vi "Read AllowUndefinedNames.vi"(9 "VisaResourceName in":refnum<class "VisaResourceName.lvclass">) -> (3 "VisaResourceName out":refnum<class "VisaResourceName.lvclass">, 4 "Allow Undefined Names":bool)   [LabVIEW 2014, in "VisaResourceName.lvclass"]
uses:
  VisaResourceName.lvclass
  VisaResourceName.lvclass/VisaResourceName.ctl
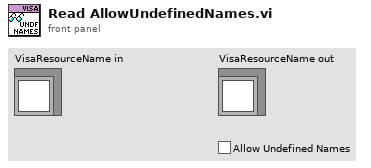
[diagram p1: front panel]
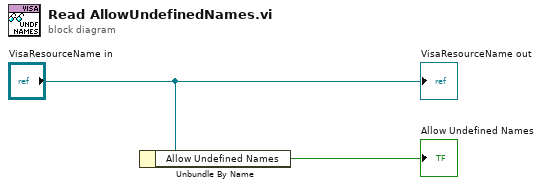
[diagram p0: block diagram]
diagram:
  n1 = Unbundle By Name("VisaResourceName in") -> ("Allow Undefined Names"=→"Allow Undefined Names":bool)
  "VisaResourceName out" <- "VisaResourceName in"
